vi "IMAQ(dx) Enumerate Cameras LV2012 NIVerified.vi"() -> (1 "Devices":string[][](table)=[["Microsoft® LifeCam Studio(TM) ", "cam2", "F5F0680977C0F2A3"]], 2 "First Resource":string, 3 "Resource":T1, 4 "# Devices":i32)   [LabVIEW 2018]
doc: "Lists connected NI-IMAQ and NI-IMAQdx cameras by querying the System Configration API and filtering for the niimaq or niimaqdx expert."
uses:
  <vilib>/userdefined/High Color/IMAQdx.ctl
  <vilib>/Utility/error.llb/DialogType.ctl
  <vilib>/nisyscfg/Close (Hardware).vi
  <vilib>/nisyscfg/Close (System).vi
  <vilib>/nisyscfg/nisyscfg.lvlib
  <resource>/objmgr/nisysapi.rc
panel:
  out "Array Size":i32[](array[numeric])
  in  "Target (localhost)":refnum<k21>="localhost"
  in  "IMAQ driver type":string(combo)="niimaqdx"
  # "Overview: Example demonstrates how to list connected NI-IMAQ and NI-IMAQdx cameras\nRequirements: LabVIEW 2012 Base Development System (or compatible)\n                             NI System Configuration API 14.0 (or compatible)\n                             NI-IMAQ 14.0 / NI-IMAQdx 14.0 (or compatible)\n\nInstructions: \n1. Select the target\n2. Select the IMAQ driver type\n3. Run the VI"
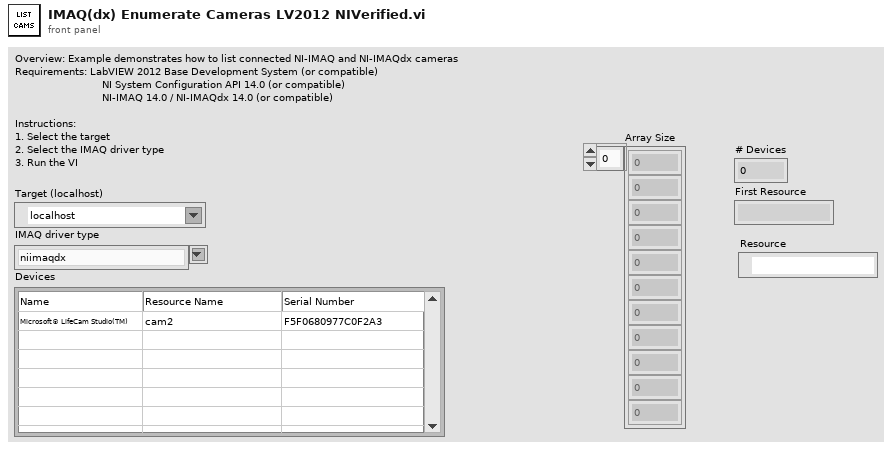
[diagram p1: front panel]
types:
  T1 = typedef "IMAQdx.ctl" = refnum<k21>
  T2 = typedef "DialogType.ctl" = u16
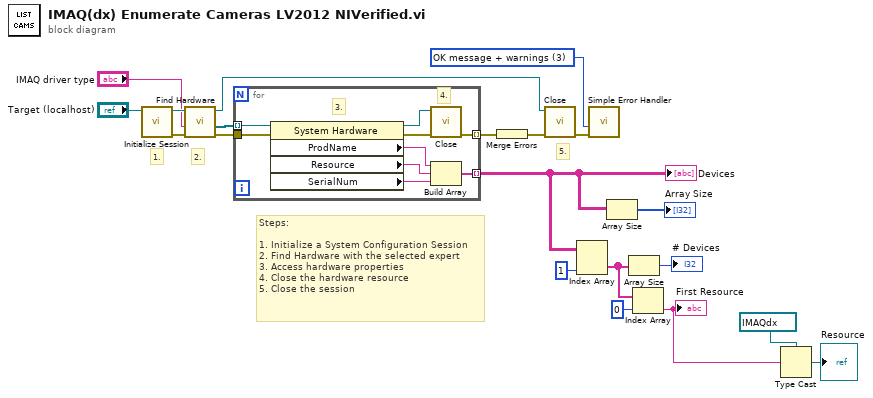
[diagram p0: block diagram]
diagram:
  w18 = T2 3 items=["no dialog", "OK message", "continue or stop message", "OK message + warnings", "continue/stop + warnings"] ("type of dialog (OK msg:1)")
  # "5."
  # "2."
  # "1."
  # "Steps:\n\n1. Initialize a System Configuration Session\n2. Find Hardware with the selected expert\n3. Access hardware properties\n4. Close the hardware resource\n5. Close the session"
  n1 = call <vilib>:"Initialize Session.vi"("Target (localhost)"="Target (localhost)") -> ("error out"=w15:errorcluster, "Session out"=w16:refnum<k21>)  [unwired: 9 in]
  n2 = call <vilib>:"Find Hardware.vi"("error in (no error)"=w15, "Experts"="IMAQ driver type", "Session in"=w16) -> ("error out"=w13:errorcluster, "Resources out"=w17:refnum<k20>[], "Session out"=w19:refnum<k21>)  [unwired: 2 in, 4 out]
  n3 = for {
    tunnel: w17 -> [w22] mode=indexing
    tunnel: [w21] -> w8 mode=indexing
    tunnel: w13 -> [w26]
    tunnel: [w29] -> w14 mode=indexing
    # "4."
    # "3."
    n4 = property class="System Hardware"(reference=w22, error in=w26) -> (reference out=w27:refnum<k20>, error out=w23:errorcluster, "ProdName"=w25:string, "Resource"=w24:string, "SerialNum"=w28:string)
    n5 = call-poly <vilib>:"Close.vi"("error in (no error)"=w23, "Resource in"=w27) -> ("error out"=w29:errorcluster)  [unwired: 9 in]
    n6 = Build Array(w25, w24, w28) -> (w21:string[])
  }
  "Devices" <- w8
  n7 = Merge Errors(w14) -> (w11:errorcluster)
  n8 = call-poly <vilib>:"Close.vi"("error in (no error)"=w11, "Session in"=w19) -> ("error out"=w20:errorcluster)  [unwired: 9 in]
  n9 = Index Array(array=w8, index (col)=1 ("disabled index (col)")) -> (element=w5:string[])  [unwired: 1 in]
  n10 = call <vilib>:"Simple Error Handler.vi"("type of dialog (OK msg:1)"=w18, "error in (no error)"=w20) -> ()  [unwired: 3 in, 5 out]
  n11 = Array Size(array=w8) -> (size(s)=→"Array Size":i32[])
  n12 = Array Size(array=w5) -> (size(s)=→"# Devices":i32)
  n13 = Index Array(array=w5, index=0) -> (element=w2:string)
  "First Resource" <- w2
  n14 = Type Cast(type=T1 "cam2" ("Select Control"), x=w2) -> (*(type *) &x=→"Resource":T1)
